vi "setUp.vi"(8 "error in (no error)":errorcluster, 11 "reference in":refnum<class "SLSC Switch Export Unit Tests.lvclass">) -> (0 "error out":errorcluster, 3 "reference out":refnum<class "SLSC Switch Export Unit Tests.lvclass">)   [LabVIEW 2017, in "SLSC Switch Export Unit Tests.lvclass"]
doc: "setUp runs prior to the test method during test execution. Use this method to initialize any object data required by your tests."
uses:
  SLSC Switch Export Unit Tests.lvclass
  C:/Program Files (x86)/National Instruments/LabVIEW 2017/vi.lib/addons/_JKI Toolkits/VI Tester/TestCase.llb/TestCase.lvclass
  NationalInstruments.VeriStand.SystemDefinitionAPI
  SLSC Switch Export Unit Tests.lvclass/SLSC Switch Export Unit Tests.ctl
  <userlib>/_OpenG.lib/file/file.llb/Append Path to Root if Relative - Scalar__ogtk.vi
  <vilib>/addons/_JKI Toolkits/VI Tester/TestCase.llb/TestCase.lvclass
  niveristand-custom-device-testing-tools/VeriStandTestUtilities/VeriStandTestUtilities.lvlib
  Shared/VeriStand SLSC Scripting/VeriStand SLSC Scripting.lvlib
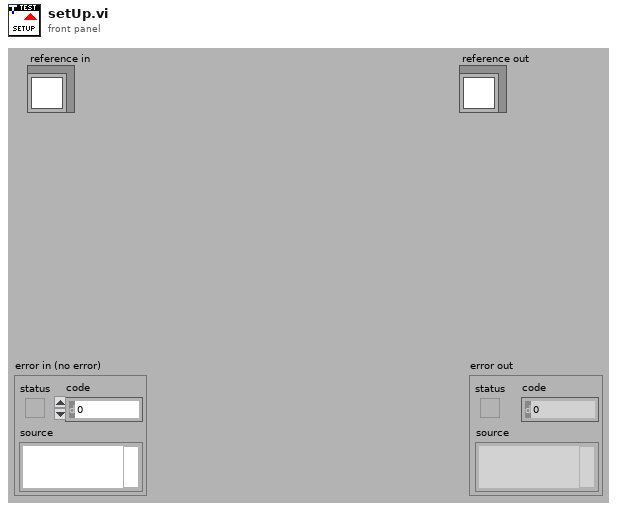
[diagram p1: front panel]
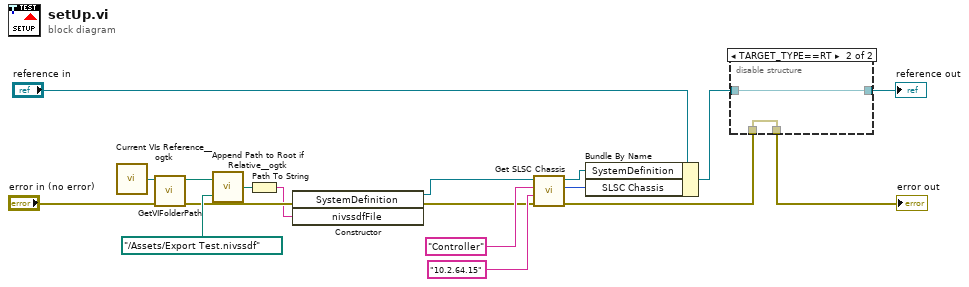
[diagram p0: block diagram]
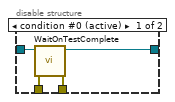
[diagram p2: hidden frame]
diagram:
  n1 = call <userlib>:"Current VIs Reference__ogtk.vi"() -> ("Current VI's reference"=w16:refnum<vi>)  [unwired: 5 in]
  n2 = call "GetVIFolderPath.vi"("error in (no error)"="error in (no error)", "VI Reference in"=w16) -> ("error out"=w12:errorcluster, "VI Folder Path out"=w15:path)  [unwired: 8 in]
  n3 = call-poly <userlib>:"Append Path to Root if Relative__ogtk.vi"("Absolute or Relative Path"=path "../Assets/Export Test.nivssdf", "Root Path"=w15) -> ("Absolute or Appended Path"=w13:path)
  n4 = Path To String(path=w13) -> (string=w11:string)
  n5 = constructor class="SystemDefinition"(error in=w12, "nivssdfFile"=w11) -> (reference out=w4:refnum<k24>, error out=w5:errorcluster)  [unwired: 2 in, 2 out]
  n6 = call "Get SLSC Chassis.vi"("error in (no error)"=w5, "SLSC Chassis Name or IP"="10.2.64.15" ("Name or IP"), "Target Name"="Controller" ("Target"), "SysDef in"=w4) -> ("error out"=w1:errorcluster, "SLSC Chassis"=w6:u64, "SysDef out"=w7:refnum<k24>)  [unwired: 4 in, 1 out]
  n7 = Bundle By Name(cluster="reference in", "SystemDefinition"=w7, "SLSC Chassis"=w6) -> (w2:refnum<class "SLSC Switch Export Unit Tests.lvclass">)
  n8 = disable-structure shown="TARGET_TYPE==RT" {
    disable-tunnel: w1 -> [w22 w23]
    disable-tunnel: [w21 w23] -> w18
    disable-tunnel: [w20 w24] -> w17
    disable-tunnel: w2 -> [w19 w24]
    frame condition #0 (active) {
      n9 = call <vilib>:"WaitOnTestComplete.vi"("error in (no error)"=w22, "TestCase in"=w19) -> ("error out"=w21:errorcluster, "TestCase out"=w20:refnum<class "SLSC Switch Export Unit Tests.lvclass">)  [unwired: 8 in]
    }
    frame condition #1 {
    }
  }
  "error out" <- w18
  "reference out" <- w17
